vi "construct.vi"(8 "error in (no error)":errorcluster, 9 "configuration name":string, 10 "load config file?":bool=TRUE, 11 "GenericPlugin in":refnum<class "StimulatorDL090503.lvclass">) -> (0 "error out":errorcluster, 3 "GenericPlugin out":refnum<class "StimulatorDL090503.lvclass">)   [LabVIEW 2010, in "StimulatorDL090503.lvclass"]
uses:
  StimulatorDL090503.lvclass
  StimulatorDL090503Scaffold/StimulatorDL090503Scaffold/StimulatorDL090503Scaffold.lvclass
  StimulatorDL090503.lvclass/StimulatorDL090503.ctl
  common/classes/GenericComponent/GenericComponent/GenericComponent.lvclass
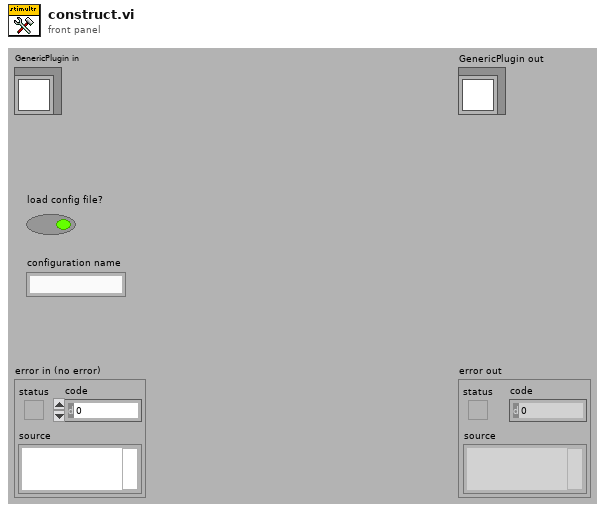
[diagram p1: front panel]
types:
  T1 = typedef "plugin_specification.ctl" = cluster{"class path":string, "configuration":string, "label":string, "settings name":string}
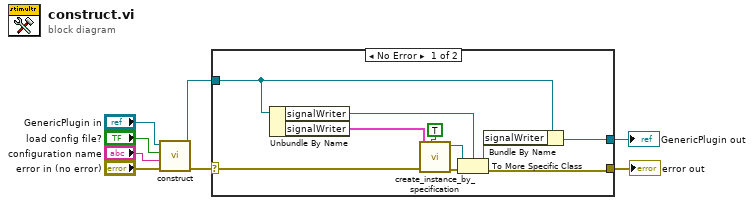
[diagram p0: block diagram]
diagram:
  n1 = call-parent "construct.vi"("error in (no error)"="error in (no error)", "configuration name"="configuration name", "load config file?"="load config file?", "GenericPlugin in"="GenericPlugin in") -> ("error out"=w3:errorcluster, "GenericPlugin out"=w2:refnum<class "StimulatorDL090503.lvclass">)  [unwired: 6 in]
  n2 = case shown="No Error" w3 {
    selector: w3 -> [w18 w20]
    tunnel: w2 -> [w11 w19]
    tunnel: [w14 w20] -> w4
    tunnel: [w9 w19] -> w1
    frame No Error {
      n3 = Unbundle By Name(w11) -> ("signalWriter"=w12:refnum<class "GenericSignalWriter.lvclass">, "signalWriter"=w13:T1)
      n4 = call "create_instance_by_specification.vi"("call constructor?"=TRUE, "error in (no error)"=w18, "component specification"=w13) -> ("error out"=w16:errorcluster, "GenericPlugin out"=w15:refnum<class "GenericComponent.lvclass">)  [unwired: 6 in, 1 out]
      n5 = To More Specific Class(target class=w12, reference=w15, error in=w16) -> (specific class reference=w10:refnum<class "GenericSignalWriter.lvclass">, error out=w14:errorcluster)
      n6 = Bundle By Name(cluster=w11, "signalWriter"=w10) -> (w9:refnum<class "StimulatorDL090503.lvclass">)
    }
    frame Error {
    }
  }
  "error out" <- w4
  "GenericPlugin out" <- w1
